vi "Get M1M3 Support Events.vi"(11 "M1M3 Support Events in":refnum<class "M1M3 Support Events.lvclass">) -> (2 "M1M3 Support Events":T1, 3 "M1M3 Support Events out":refnum<class "M1M3 Support Events.lvclass">)   [LabVIEW 2016, in "M1M3 Support Events.lvclass"]
uses:
  M1M3 Support Events.lvclass
  Typedefs/M1M3 Support Events.ctl
  SALLV_m1m3/DataTypes/InclinometerData.ctl
  SALLV_m1m3/DataTypes/IMSData.ctl
  Typedefs/SAL Connected.ctl
  SALLV_m1m3/DataTypes/AccelerometerData.ctl
  SALLV_m1m3/DataTypes/OuterLoopData.ctl
  SALLV_m1m3/DataTypes/logevent_ErrorCode.ctl
  SALLV_m1m3/DataTypes/logevent_InterlockStatus.ctl
  SALLV_m1m3/DataTypes/logevent_InterlockWarning.ctl
  SALLV_m1m3/DataTypes/GyroData.ctl
  SALLV_m1m3/DataTypes/logevent_HardpointActuatorInfo.ctl
  SALLV_m1m3/DataTypes/logevent_ForceActuatorInfo.ctl
  SALLV_m1m3/DataTypes/logevent_HardpointMonitorInfo.ctl
  SALLV_m1m3/DataTypes/ForceActuatorData.ctl
  SALLV_m1m3/DataTypes/HardpointActuatorData.ctl
  SALLV_m1m3/DataTypes/HardpointMonitorData.ctl
  SALLV_m1m3/DataTypes/logevent_AirSupplyStatus.ctl
  SALLV_m1m3/DataTypes/logevent_AirSupplyWarning.ctl
  SALLV_m1m3/DataTypes/PowerSupplyData.ctl
  SALLV_m1m3/DataTypes/PIDData.ctl
  SALLV_m1m3/DataTypes/logevent_PIDInfo.ctl
  SALLV_m1m3/DataTypes/logevent_PowerStatus.ctl
  SALLV_m1m3/DataTypes/logevent_PowerSupplyStatus.ctl
  SALLV_m1m3/DataTypes/logevent_PowerWarning.ctl
  SALLV_m1m3/DataTypes/logevent_SummaryState.ctl
  SALLV_m1m3/DataTypes/logevent_DetailedState.ctl
  SALLV_m1m3/DataTypes/logevent_ForceActuatorForceWarning.ctl
  SALLV_m1m3/DataTypes/logevent_ForceActuatorWarning.ctl
  SALLV_m1m3/DataTypes/logevent_ForceActuatorState.ctl
  SALLV_m1m3/DataTypes/logevent_AppliedAberrationForces.ctl
  SALLV_m1m3/DataTypes/logevent_AppliedAccelerationForces.ctl
  SALLV_m1m3/DataTypes/logevent_AppliedAzimuthForces.ctl
  SALLV_m1m3/DataTypes/logevent_AppliedActiveOpticForces.ctl
  SALLV_m1m3/DataTypes/logevent_AppliedBalanceForces.ctl
  SALLV_m1m3/DataTypes/logevent_AppliedCylinderForces.ctl
  SALLV_m1m3/DataTypes/logevent_AppliedElevationForces.ctl
  SALLV_m1m3/DataTypes/logevent_AppliedForces.ctl
  SALLV_m1m3/DataTypes/logevent_AppliedOffsetForces.ctl
  SALLV_m1m3/DataTypes/logevent_AppliedStaticForces.ctl
  SALLV_m1m3/DataTypes/logevent_AppliedThermalForces.ctl
  SALLV_m1m3/DataTypes/logevent_AppliedVelocityForces.ctl
  SALLV_m1m3/DataTypes/logevent_RejectedAberrationForces.ctl
  SALLV_m1m3/DataTypes/logevent_RejectedAccelerationForces.ctl
  SALLV_m1m3/DataTypes/logevent_RejectedActiveOpticForces.ctl
  SALLV_m1m3/DataTypes/logevent_RejectedAzimuthForces.ctl
  SALLV_m1m3/DataTypes/logevent_RejectedBalanceForces.ctl
  SALLV_m1m3/DataTypes/logevent_RejectedCylinderForces.ctl
  SALLV_m1m3/DataTypes/logevent_RejectedElevationForces.ctl
  SALLV_m1m3/DataTypes/logevent_RejectedForces.ctl
  SALLV_m1m3/DataTypes/logevent_RejectedOffsetForces.ctl
  SALLV_m1m3/DataTypes/logevent_RejectedStaticForces.ctl
  SALLV_m1m3/DataTypes/logevent_RejectedThermalForces.ctl
  SALLV_m1m3/DataTypes/logevent_RejectedVelocityForces.ctl
  SALLV_m1m3/DataTypes/logevent_CommandRejectionWarning.ctl
  SALLV_m1m3/DataTypes/logevent_SettingVersions.ctl
  SALLV_m1m3/DataTypes/logevent_SettingsApplied.ctl
  SALLV_m1m3/DataTypes/logevent_HardpointActuatorState.ctl
  SALLV_m1m3/DataTypes/logevent_HardpointActuatorWarning.ctl
  SALLV_m1m3/DataTypes/logevent_HardpointMonitorState.ctl
  SALLV_m1m3/DataTypes/logevent_HardpointMonitorWarning.ctl
  SALLV_m1m3/DataTypes/logevent_AccelerometerWarning.ctl
  SALLV_m1m3/DataTypes/logevent_AppliedSettingsMatchStart.ctl
  SALLV_m1m3/DataTypes/logevent_CellLightStatus.ctl
  SALLV_m1m3/DataTypes/logevent_CellLightWarning.ctl
  SALLV_m1m3/DataTypes/logevent_DisplacementSensorWarning.ctl
  SALLV_m1m3/DataTypes/logevent_ForceSetpointWarning.ctl
  SALLV_m1m3/DataTypes/logevent_GyroWarning.ctl
  SALLV_m1m3/DataTypes/logevent_ILCWarning.ctl
  SALLV_m1m3/DataTypes/logevent_InclinometerSensorWarning.ctl
  M1M3 Support Events.lvclass/M1M3 Support Events.ctl
  Typedefs/M1M3SupportEUI_TypeDefs.lvlib
  SALLV_m1m3/SALLV_m1m3.lvlib
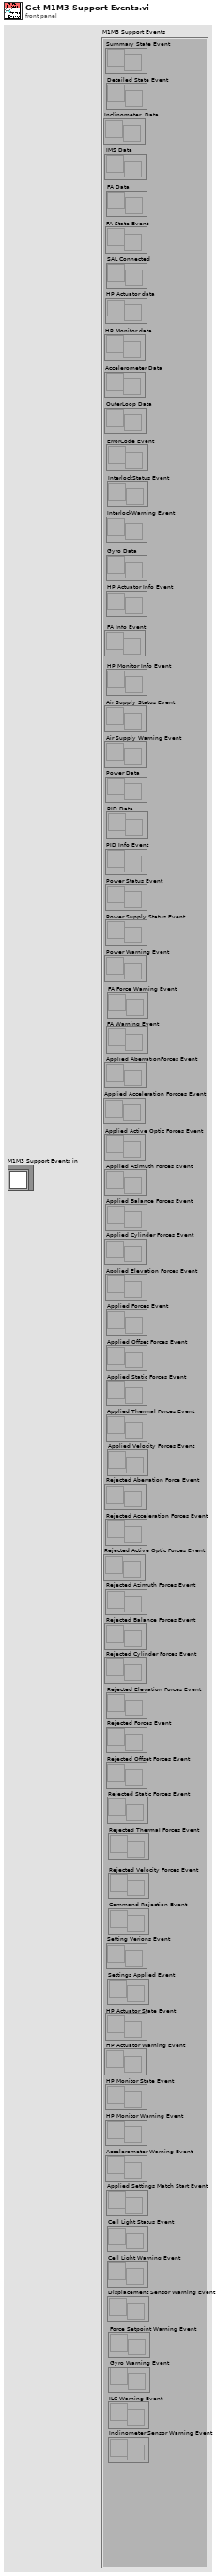
[diagram p1: front panel]
types:
  T1 = typedef "M1M3SupportEUI_TypeDefs.lvlib/M1M3 Support Events.ctl" = cluster{"Inclinometer  Data":refnum<user-event>, "IMS Data":refnum<user-event>, "SAL Connected":refnum<user-event>, "Accelerometer Data":refnum<user-event>, "OuterLoop Data":refnum<user-event>, "ErrorCode Event":refnum<user-event>, "InterlockStatus Event":refnum<user-event>, "InterlockWarning Event":refnum<user-event>, "Gyro Data":refnum<user-event>, "HP Actuator Info Event":refnum<user-event>, " FA Info Event":refnum<user-event>, "HP Monitor Info Event":refnum<user-event>, "FA Data":refnum<user-event>, "HP Actuator data":refnum<user-event>, "HP Monitor data":refnum<user-event>, "Air Supply Status Event":refnum<user-event>, "Air Supply Warning Event":refnum<user-event>, "Power Data":refnum<user-event>, "PID Data":refnum<user-event>, "PID Info Event":refnum<user-event>, "Power Status Event":refnum<user-event>, "Power Supply Status Event":refnum<user-event>, "Power Warning Event":refnum<user-event>, "Summary State Event":refnum<user-event>, "Detailed State Event":refnum<user-event>, "FA Force Warning Event":refnum<user-event>, "FA Warning Event":refnum<user-event>, "FA State Event":refnum<user-event>, "Applied AberrationForces Event":refnum<user-event>, "Applied Acceleration Forcces Event":refnum<user-event>, "Applied Azimuth Forces Event":refnum<user-event>, "Applied Active Optic Forces Event":refnum<user-event>, "Applied Balance Forces Event":refnum<user-event>, "Applied Cylinder Forces Event":refnum<user-event>, "Applied Elevation Forces Event":refnum<user-event>, "Applied Forces Event":refnum<user-event>, "Applied Offset Forces Event":refnum<user-event>, "Applied Static Forces Event":refnum<user-event>, "Applied Thermal Forces Event":refnum<user-event>, "Applied Velocity Forces Event":refnum<user-event>, "Rejected Aberration Force Event":refnum<user-event>, "Rejected Acceleration Forces Event":refnum<user-event>, "Rejected Active Optic Forces Event":refnum<user-event>, "Rejected Azimuth Forces Event":refnum<user-event>, "Rejected Balance Forces Event":refnum<user-event>, "Rejected Cylinder Forces Event":refnum<user-event>, "Rejected Elevation Forces Event":refnum<user-event>, "Rejected Forces Event":refnum<user-event>, "Rejected Offset Forces Event":refnum<user-event>, "Rejected Static Forces Event":refnum<user-event>, "Rejected Thermal Forces Event":refnum<user-event>, "Rejected Velocity Forces Event":refnum<user-event>, "Command Rejection Event":refnum<user-event>, "Setting Verions Event":refnum<user-event>, "Settings Applied Event":refnum<user-event>, "HP Actuator State Event":refnum<user-event>, "HP Actuator Warning Event":refnum<user-event>, "HP Monitor State Event":refnum<user-event>, "HP Monitor Warning Event":refnum<user-event>, "Accelerometer Warning Event":refnum<user-event>, "Applied Settings Match Start Event":refnum<user-event>, "Cell Light Status Event ":refnum<user-event>, "Cell Light Warning Event":refnum<user-event>, "Displacement Sensor Warning Event":refnum<user-event>, "Force Setpoint Warning Event":refnum<user-event>, "Gyro Warning Event ":refnum<user-event>, "ILC Warning Event ":refnum<user-event>, "Inclinometer Sensor Warning Event ":refnum<user-event>}
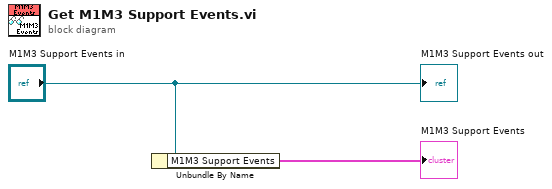
[diagram p0: block diagram]
diagram:
  n1 = Unbundle By Name("M1M3 Support Events in") -> ("M1M3 Support Events"=→"M1M3 Support Events":T1)
  "M1M3 Support Events out" <- "M1M3 Support Events in"
